vi "GetNowDateTimeString.vi"() -> (0 "时间字符串":string)   [LabVIEW 2018]
uses:
  <vilib>/addons/database/Auxilliary.llb/DB Tools Format Datetime String (Time Stamp).vi
  <vilib>/addons/database/NI_Database_API.lvlib
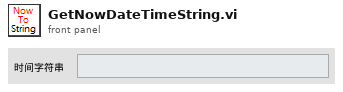
[diagram p1: front panel]
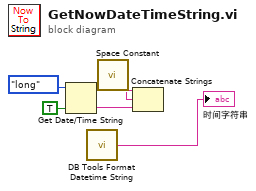
[diagram p0: block diagram]
diagram:
  n1 = Get Date/Time String(date format (0)=enum16{"short", "long", "abbreviated"}."long" ("日期格式(0)"), want seconds? (F)=TRUE ("需要秒？(F)")) -> (date string=w4:string, time string=w3:string)  [unwired: 1 in]
  n2 = call-poly <vilib>:"DB Tools Format Datetime String.vi"() -> ("date/time string"=→"时间字符串":string)  [unwired: 1 in]
  n3 = call <vilib>:"Space Constant.vi"() -> ("String"=w2:string)
  n4 = Concatenate Strings(w4, w2, w3) -> ()  [unwired: 1 out]
